vi "Comfirm Correct UserName and Password.vi"(8 "error in (no error)":errorcluster, 9 "Password":string, 10 "UserName":string) -> (0 "error out":errorcluster, 1 "Password out":string, 2 "UserName out":string, 3 "ok？":bool)   [LabVIEW 2014]
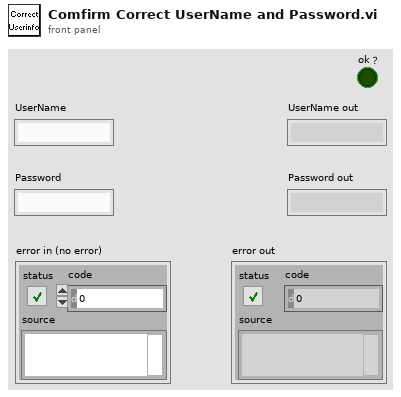
[diagram p1: front panel]
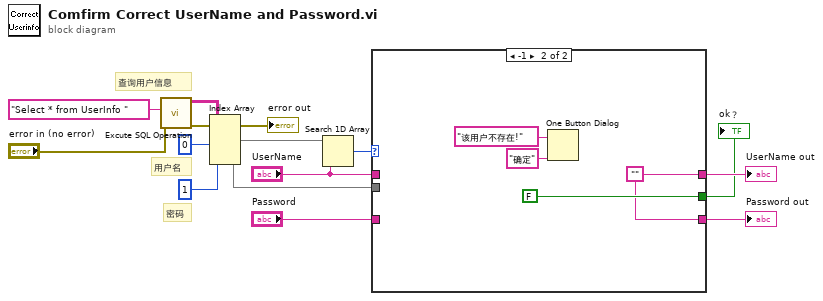
[diagram p0: block diagram]
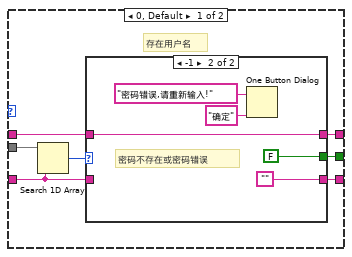
[diagram p2: hidden frame]
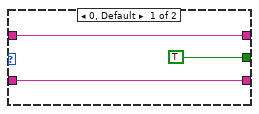
[diagram p3: hidden frame]
diagram:
  # "密码"
  # "用户名"
  # "查询用户信息"
  n1 = call "Excute SQL Operation.vi"("error in (no error)"="error in (no error)", "Cmd Text"="Select * from UserInfo ") -> ("error out"=→"error out":errorcluster, "2D-Data"=w13:string[][])  [unwired: 7 in, 1 out]
  n2 = Index Array(array=w13, index (col) #1=0 ("disabled index (col)"), index (col) #2=1 ("disabled index (col)")) -> (element #1=w10:string[], element #2=w8:string[])  [unwired: 2 in]
  n3 = Search 1D Array(1D array=w10, element="UserName") -> (index of element=w9:i32)  [unwired: 1 in]
  n4 = case shown="-1" w9 {
    tunnel: w8 -> [w21 _]
    tunnel: "Password" -> [w18 _]
    tunnel: [w19 FALSE] -> w3
    tunnel: [w17 w30] -> w6
    tunnel: "UserName" -> [w16 _]
    tunnel: [w15 w30] -> w4
    frame 0, Default {
      # "存在用户名"
      n5 = Search 1D Array(1D array=w21, element=w18) -> (index of element=w20:i32)  [unwired: 1 in]
      n6 = case shown="-1" w20 {
        tunnel: [TRUE FALSE] -> w19
        tunnel: w18 -> [w23 _]
        tunnel: [w23 ""] -> w17
        tunnel: w16 -> [w22 w26]
        tunnel: [w22 w26] -> w15
        frame 0, Default {
        }
        frame -1 {
          # "密码不存在或密码错误"
          n7 = One Button Dialog(message="密码错误,请重新输入!", button name ("OK")="确定") -> ()  [unwired: 1 out]
        }
      }
    }
    frame -1 {
      w30 = ""
      n8 = One Button Dialog(message="该用户不存在!", button name ("OK")="确定") -> ()  [unwired: 1 out]
    }
  }
  "UserName out" <- w4
  "Password out" <- w6
  "ok？" <- w3
